vi "Test SenseHat Fill.vi"() -> ()   [LabVIEW 2020]
uses:
  <vilib>/MakerHub/LINX/LMH-LINX.lvlib
  src/RPI.SenseHat.Display/Classes/SenseHat.Display/RPI.SenseHat.Display.lvclass
  <vilib>/MakerHub/LINX/Public/Utilities/Open Local.vi
  src/RPI.SenseHat.Display/Classes/Color/Color.lvclass
panel:
  in  "Color Box":u32(colorbox)
  out "Device Name":string
  out "Error Out":errorcluster
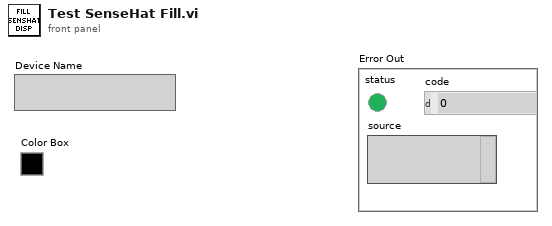
[diagram p1: front panel]
types:
  T1 = typedef "LMH-LINX.lvlib/LINX Ref.ctl" = cluster{"IO":T2, "Interface":T3, "LINX Device Config":T4}
  T2 = typedef "LMH-LINX.lvlib/Platform.ctl" = enum16{"Remote", "Local"}
  T3 = typedef "LMH-LINX.lvlib/Interface.ctl" = enum16{"Serial", "TCP"}
  T4 = typedef "LMH-LINX.lvlib/Device.lvlib/LINX Device Config.ctl" = cluster{"Interface":T3, "COM Port":refnum<visa-resource-name>, "TCP Configuration":T5, "Device Family":u8, "Device ID":u8, "Device Name":string, "TCP Ref":refnum<k5>, "Channels":T6}
  T5 = typedef "LMH-LINX.lvlib/Device.lvlib/TCP Config.ctl" = cluster{"IP Address":string, "Port":u16}
  T6 = typedef "LMH-LINX.lvlib/Channels.ctl" = cluster{"DI":u8[], "DO":u8[], "AI":u8[], "AO":u8[], "PWM":u8[], "QE":u8[], "UART":u8[], "I2C 2":u8[], "SPI":u8[], "CAN":u8[], "Servo":u8[], "AI Ref (V)":dbl, "AI Resolution (Bits)":u8, "AO Ref (V)":dbl, "AO Resolution (Bits)":u8}
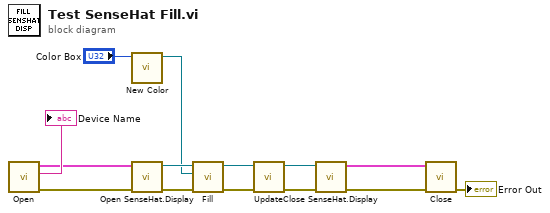
[diagram p0: block diagram]
diagram:
  n1 = call-poly <vilib>:"Open.vi"() -> ("Error Out"=w12:errorcluster, "Device Name"=→"Device Name":string, "LINX Resource"=w5:T1)  [unwired: 9 in]
  n2 = call "New Color.vi"("Color Box"="Color Box") -> ("Color out"=w2:refnum<class "Color.lvclass">)  [unwired: 9 in, 1 out]
  n3 = call "Open SenseHat.Display.vi"("error in (no error)"=w12, "LINX Resource"=w5) -> ("error out"=w11:errorcluster, "senseHatDisplay out"=w10:refnum<class "RPI.SenseHat.Display.lvclass">)  [unwired: 8 in]
  n4 = call "Fill.vi"("error in (no error)"=w11, "Color"=w2, "senseHatDisplay in"=w10) -> ("error out"=w4:errorcluster, "senseHatDisplay out"=w3:refnum<class "RPI.SenseHat.Display.lvclass">)  [unwired: 7 in]
  n5 = call "Update.vi"("error in (no error)"=w4, "senseHatDisplay in"=w3) -> ("error out"=w8:errorcluster, "senseHatDisplay out"=w9:refnum<class "RPI.SenseHat.Display.lvclass">)  [unwired: 8 in]
  n6 = call "Close SenseHat.Display.vi"("error in (no error)"=w8, "senseHatDisplay in"=w9) -> ("error out"=w13:errorcluster, "LINX Resource"=w14:T1)  [unwired: 8 in]
  n7 = call <vilib>:"Close.vi"("Error In"=w13, "LINX Resource"=w14) -> ("Error Out"=→"Error Out":errorcluster)  [unwired: 9 in]
